vi "bang.vi"(6 "Sanity":dbl, 7 "Start":bool, 8 "Tolerance":dbl, 10 "Set":dbl, 11 "Pos":dbl) -> (2 "B_Out":bool)   [LabVIEW 2013]
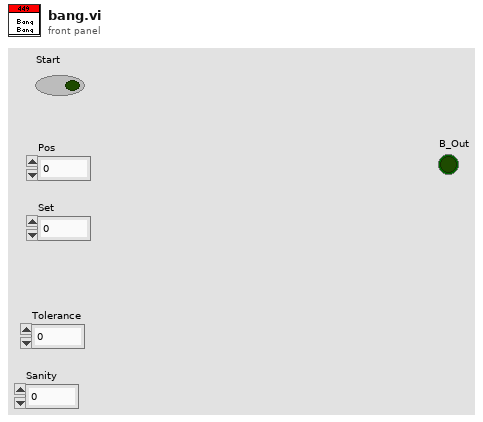
[diagram p1: front panel]
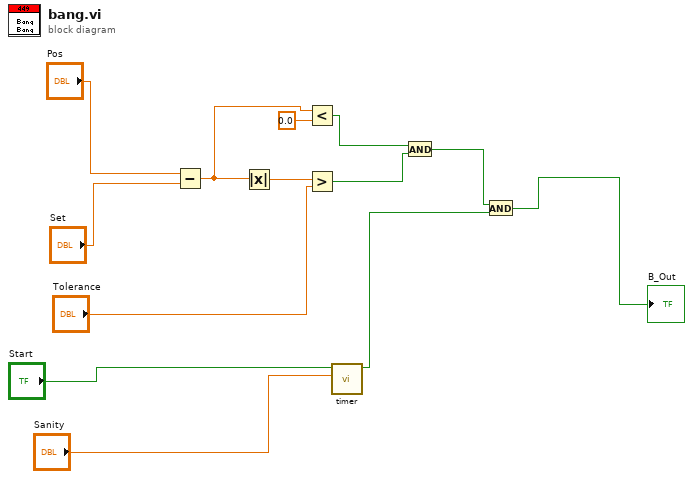
[diagram p0: block diagram]
diagram:
  n1 = Subtract(x="Pos", y="Set") -> (x-y=w8:dbl)
  n2 = Absolute Value(x=w8) -> (abs(x)=w11:dbl)
  n3 = Less?(x=w8, y=0.0) -> (x < y?=w7:bool)
  n4 = Greater?(x=w11, y="Tolerance") -> (0:w6:bool)
  n5 = call "timer.vi"("Time"="Sanity", "Set"="Start") -> ("Out"=w3:bool)  [unwired: 9 in]
  n6 = And(x=w7, y=w6) -> (x .and. y?=w4:bool)
  n7 = And(x=w4, y=w3) -> (x .and. y?=→"B_Out":bool)
